vi "occupancy_grid.vi"(0 "Occupancy Grid configuration":string="{\n     \"type\": \"OccupancyGrid\",\n     \"listen_port\": 8015,\n     \"stream_dimensions\": {\n       \"x\": 512.0,\n       \"y\": 512.0\n     },\n    \"meters_per_pixel\": 0.1,\n    \"follow_yaw\":  false,\n    \"follow_pitch\": false,\n    \"follow_roll\": false,\n    \"ray_tracing\":{\n        \"enable_ray_tracing\": false\n     },\n    \"annotation\": {\n      \"include_annotation\": false,\n      \"desired_tags\": [\n        \"traffic_sign\", \"vehicle\"\n      ],\n      \"far_plane\": 10000.0,\n      \"include_tags\": true,\n      \"include_obb\": false\n    }\n}", 3 "error In":errorcluster) -> (4 "Camera configuration":string, 6 "Annotated Image":picture, 7 "Raw data":u8[](array[numeric]), 8 "Annotation Data":string, 9 "error out":errorcluster)   [LabVIEW 2019]
doc: "Configures and reads the data stream for an Occupancy Grid sensor and outputs a picture of the specified size on the configuration."
uses:
  controls/Header.ctl
  tools/simx_common.vi
panel:
  out "Header":T1 {"game_time" format="%_10g"}
  in  "null connection":refnum<k5>
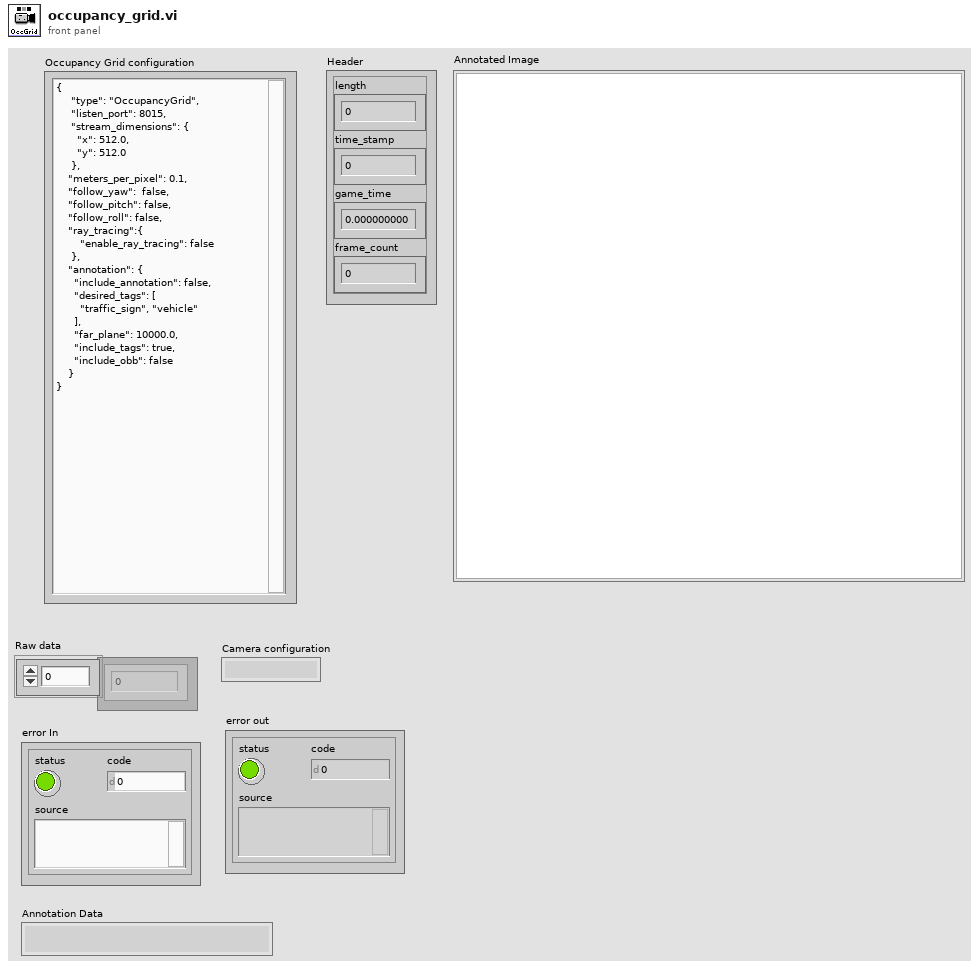
[diagram p1: front panel]
types:
  T1 = typedef "Header.ctl" = cluster{"length":u32, "time_stamp":u32, "game_time":sgl, "frame_count":u32}
  T2 = typedef "simx_connection.ctl" = cluster{"Config":T3, "Connections":T6, "Map":cluster{"lanes":cluster{"x":dbl[], "y":dbl[], "z":dbl[]}, "StartPosition":cluster{"start_points":T7, "StartRotation":dbl[], "StartLocation":dbl[]}, "Draw Map Size":T8, "DrawArea":cluster{"min_Y":dbl, "min_X":dbl, "Scale X":dbl, "Scale Y":dbl}, "Map":picture, "Map Geojson":string}}
  T3 = typedef "config.ctl" = cluster{"Trajectory":T4, "Weather":T5}
  T4 = typedef "trajectory.ctl" = cluster{"Number of frames":i32, "Frame number":i32, "Trajectory":string}
  T5 = typedef "weather.ctl" = cluster{"id":string}
  T6 = typedef "connections.ctl" = cluster{"Simulator Connection":refnum<k5>, "server_ip":string, "Port":i32, "Sensor connections":refnum<k5>[]}
  T7 = typedef "start_points.ctl" = cluster{"locations":dbl[][], "rotations":dbl[][], "type":string[]}
  T8 = typedef "LVBoundsTypeDef.ctl" = cluster{"Width":u32, "Height":u32}
  T9 = typedef "sensor_sample.ctl" = cluster{"Header":T1, "data out":string}
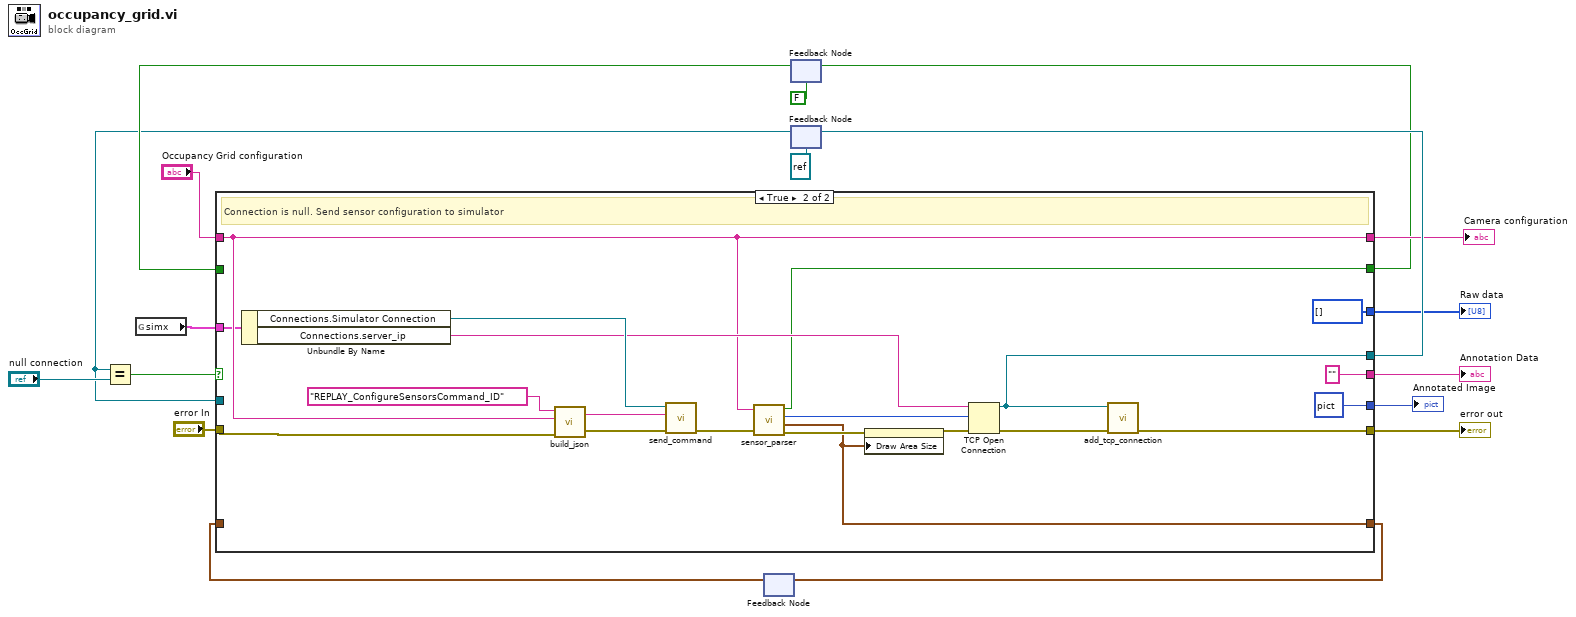
[diagram p0: block diagram]
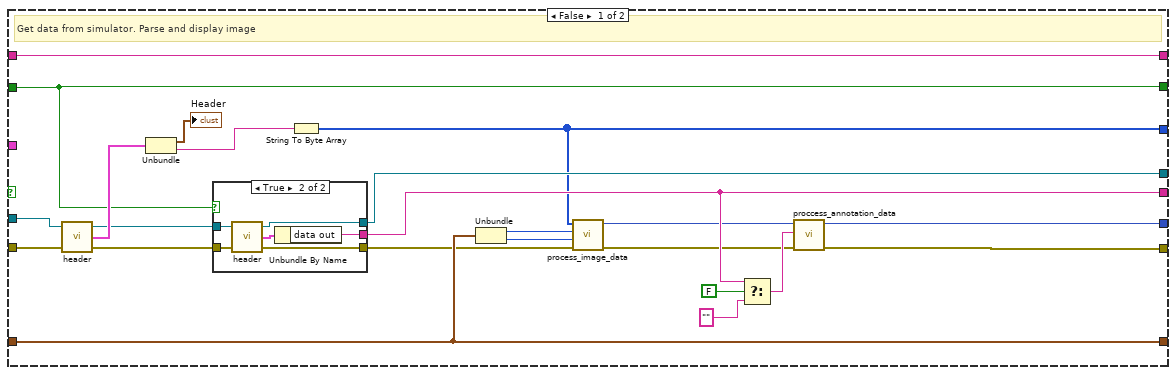
[diagram p2: hidden frame]
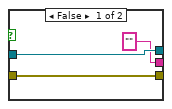
[diagram p3: hidden frame]
diagram:
  n1 = global read "simx_common.vi" "simx"() -> (w3:T2)
  n2 = feedback #1() -> (w11:cluster{"x dimension":i32, "y dimension":i32})  [unwired: 1 in]
  n3 = feedback #2(FALSE) -> (w5:bool)
  n4 = feedback #3(refnum<k5> refnum ("connection ID")) -> (w2:refnum<k5>)
  n5 = Equal?(x=w2, y="null connection") -> (x = y?=w15:bool)
  n6 = case shown="True" w15 {
    tunnel: [w34 w51] -> w14
    tunnel: "Occupancy Grid configuration" -> [w36 w55]
    tunnel: [w26 w53] -> w16
    tunnel: w2 -> [w39 _]
    tunnel: "error In" -> [w38 w61]
    tunnel: w11 -> [w37 _]
    tunnel: [w33 picture data[5B] ("new picture")] -> w8
    tunnel: [w37 w58] -> w12
    tunnel: [w22 u8[] [] ("unsigned byte array")] -> w10
    tunnel: [w36 w55] -> w9
    tunnel: [w35 w57] -> w7
    tunnel: w5 -> [w35 _]
    tunnel: [w32 "" ("data out")] -> w4
    tunnel: w3 -> [_ w54]
    frame False {
      # "Get data from simulator. Parse and display image"
      n7 = call "header.vi"("error in"=w38, "TCP Network Connection in"=w39) -> ("error out"=w23:errorcluster, "Sensor sample"=w40:T9, "TCP Network Connection out"=w30:refnum<k5>)  [unwired: 1 in]
      n8 = Unbundle(w40) -> ("Header"=→"Header":T1, "data out"=w41:string)
      n9 = case shown="True" w35 {
        tunnel: w30 -> [w44 w50]
        tunnel: [w44 w49] -> w26
        tunnel: w23 -> [w42 w48]
        tunnel: ["" ("data out") w46] -> w32
        tunnel: [w42 w45] -> w25
        frame False {
        }
        frame True {
          n10 = call "header.vi"("error in"=w48, "TCP Network Connection in"=w50) -> ("error out"=w45:errorcluster, "Sensor sample"=w47:T9, "TCP Network Connection out"=w49:refnum<k5>)  [unwired: 1 in]
          n11 = Unbundle By Name(w47) -> ("data out"=w46:string)
        }
      }
      n12 = String To Byte Array(string=w41) -> (unsigned byte array=w22:u8[])
      n13 = Unbundle(w37) -> ("x dimension"=w21:i32, "y dimension"=w20:i32)
      n14 = call "process_image_data.vi"("error in"=w25, "y"=w20, "x"=w21, "Raw data"=w22) -> ("error out"=w24:errorcluster, "Image"=w19:picture)  [unwired: 4 in]
      n15 = Select(t=w32, s=FALSE ("Show Annotation"), f="") -> (s? t:f=w27:string)
      n16 = call "proccess_annotation_data.vi"("error in"=w24, "Annotation Data"=w27, "Image in"=w19) -> ("error out"=w34:errorcluster, "Image out"=w33:picture)  [unwired: 2 in, 1 out]
    }
    frame True {
      # "Connection is null. Send sensor configuration to simulator"
      n17 = Unbundle By Name(w54) -> ("Connections.Simulator Connection"=w64:refnum<k5>, "Connections.server_ip"=w62:string)
      n18 = call "build_json.vi"("error in"=w61, "Message"=w55, "Command_ID"="REPLAY_ConfigureSensorsCommand_ID") -> ("error out"=w68:errorcluster, "JSON Out"=w69:string)  [unwired: 1 in]
      n19 = call "send_command.vi"("error in"=w68, "JSON Command"=w69, "TCP Network Connection in"=w64) -> ("error out"=w60:errorcluster)  [unwired: 1 in, 3 out]
      n20 = call "sensor_parser.vi"("Sensor configuration"=w55, "error in"=w60) -> ("include_annotation"=w57:bool, "Port out"=w56:u16, "Stream dimensions"=w58:cluster{"x dimension":i32, "y dimension":i32}, "error out"=w59:errorcluster)  [unwired: 1 in]
      n21 = property on="Annotated Image" class="Pict"(error in=w59, "Draw Area Size"=w58) -> (error out=w63:errorcluster)  [unwired: 1 in, 1 out]
      n22 = TCP Open Connection(address=w62, remote port or service name=w56, error in (no error)=w63) -> (connection ID=w53:refnum<k5>, error out=w52:errorcluster)  [unwired: 2 in]
      n23 = call "add_tcp_connection.vi"("error in"=w52, "Sensor connection"=w53) -> ("error out"=w51:errorcluster)  [unwired: 5 in]
    }
  }
  "error out" <- w14
  "Annotated Image" <- w8
  "Raw data" <- w10
  "Camera configuration" <- w9
  "Annotation Data" <- w4
  n24 = feedback-in #1(w12) -> ()
  n25 = feedback-in #2(w7) -> ()
  n26 = feedback-in #3(w16) -> ()
